vi "Self Test.vi"(8 "error in":errorcluster, 11 "69X_79X in":refnum<class "79XRP.lvclass">) -> (0 "error out":errorcluster, 3 "69X_79X out":refnum<class "79XRP.lvclass">)   [LabVIEW 2019, in "79XRP.lvlib" / "79XRP.lvclass"]
uses:
  Library/79XRP.lvclass
  Library/79XRP.lvclass/79XRP.ctl
  builds/Instruments/PowerSupply.lvlibp/Library/PowerSupply.lvclass
  <instrlib>/Keysight RP7900 Series/Keysight RP7900 Series.lvlib
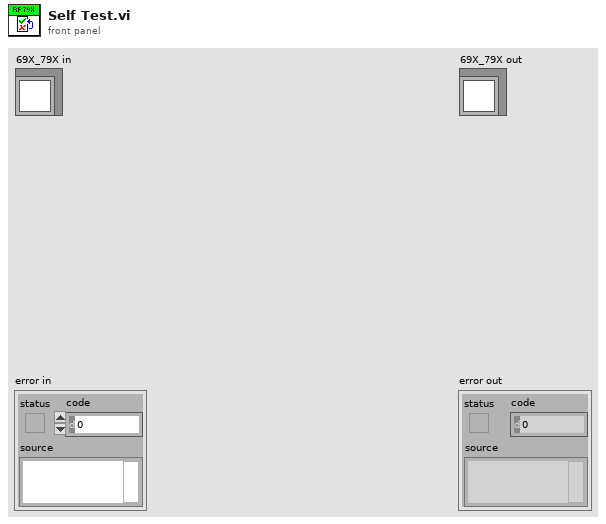
[diagram p1: front panel]
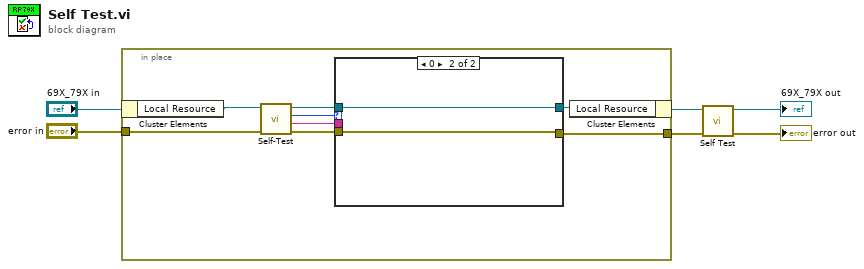
[diagram p0: block diagram]
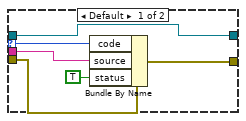
[diagram p2: hidden frame]
diagram:
  n1 = in-place {
    in-place-border: "error in" -> [w8]
    in-place-border: [w13] -> w2
    n2 = in-place-cluster #1("69X_79X in") -> ("Local Resource"=w7:refnum<visa-resource-name>)
    n3 = call <instrlib>:"Self-Test.vi"("error in (no error)"=w8, "VISA resource name"=w7) -> ("error out"=w9:errorcluster, "Self-Test Result Message"=w10:string, "Self-Test Result Code"=w11:i32, "VISA resource name out"=w12:refnum<visa-resource-name>)  [unwired: 6 in]
    n4 = case shown="0" w11 {
      selector: w11 -> [w19 _]
      tunnel: w12 -> [w15 w21]
      tunnel: w9 -> [w20 w22]
      tunnel: w10 -> [w18 _]
      tunnel: [w16 w22] -> w13
      tunnel: [w15 w21] -> w14
      frame Default {
        n5 = Bundle By Name(cluster=w20, "code"=w19, "source"=w18, "status"=TRUE) -> (w16:errorcluster)
      }
      frame 0 {
      }
    }
    n6 = in-place-cluster #1("Local Resource"=w14) -> (w4:refnum<class "79XRP.lvclass">)
  }
  n7 = call-parent "Self Test.vi"("error in"=w2, "Instruments in"=w4) -> ("error out"=→"error out":errorcluster, "Instruments out"=→"69X_79X out":refnum<class "79XRP.lvclass">)  [unwired: 8 in]
